vi "Open config file.vi"(8 "error in (no error)":errorcluster, 11 "MAG config file path":path) -> (0 "error out":errorcluster, 1 "cancelled prompt":bool, 2 "prompted":bool, 3 "Refnum out":T1)   [LabVIEW 2024]
doc: "Opens config file and returns its refnum.\nIf file cannot be found, user will be prompt to select configuration file."
uses:
  <vilib>/Utility/config.llb/Config Data RefNum.ctl
  <vilib>/Utility/config.llb/NI_LVConfig.lvlib
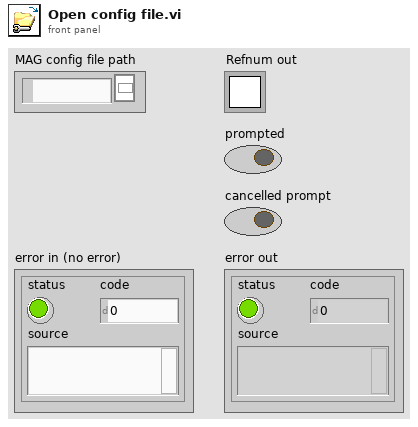
[diagram p1: front panel]
types:
  T1 = typedef "NI_LVConfig.lvlib/Config Data RefNum.ctl" = refnum<k1>
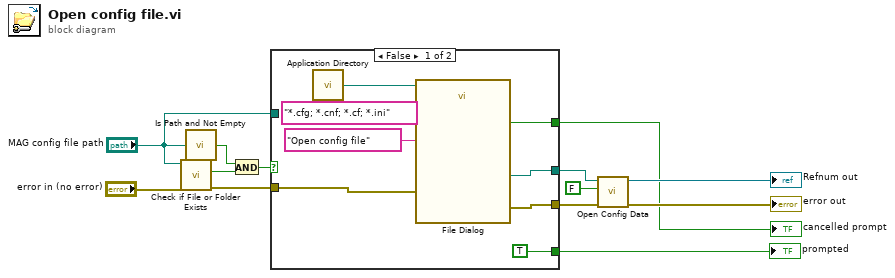
[diagram p0: block diagram]
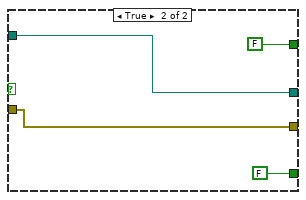
[diagram p2: hidden frame]
diagram:
  n1 = call <vilib>:"Check if File or Folder Exists.vi"("error in (no error)"="error in (no error)", "path"="MAG config file path") -> ("error out"=w6:errorcluster, "file or folder exists?"=w9:bool)  [unwired: 7 in, 1 out]
  n2 = call <vilib>:"Is Path and Not Empty.vi"("path"="MAG config file path") -> ("Is Path and Not Empty?"=w11:bool)  [unwired: 4 in]
  n3 = And(x=w11, y=w9) -> (x .and. y?=w10:bool)
  n4 = case shown="False" w10 {
    tunnel: [w19 w25] -> w3
    tunnel: "MAG config file path" -> [_ w25]
    tunnel: [w18 w24] -> w4
    tunnel: w6 -> [w17 w24]
    tunnel: [TRUE FALSE] -> w13
    tunnel: [w14 FALSE ("cancelled")] -> w1
    frame False {
      n5 = call <vilib>:"Application Directory.vi"() -> ("Application Directory"=w16:path)
      n6 = call "File Dialog"("start path"=w16, "prompt"="Open config file" ("default name"), "error in"=w17, "pattern (all files)"="*.cfg; *.cnf; *.cf; *.ini") -> ("selected path"=w19:path, "cancelled"=w14:bool, "error out"=w18:errorcluster)  [unwired: 8 in, 1 out]
    }
    frame True {
    }
  }
  "cancelled prompt" <- w1
  "prompted" <- w13
  n7 = call <vilib>:"Open Config Data.vi"("error in (no error)"=w4, "create file if necessary (T)"=FALSE, "configuration file path"=w3) -> ("error out"=→"error out":errorcluster, "refnum"=→"Refnum out":T1)  [unwired: 6 in, 1 out]
